vi "state change.vi"(11 "game state":T1(ring)) -> (3 "T/F":bool)   [LabVIEW 2023]
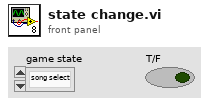
[diagram p1: front panel]
types:
  T1 = enum16{"song select", "difficulty select", "gameplay", "result"}
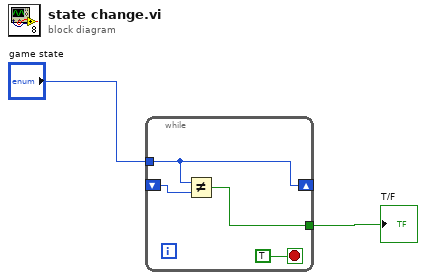
[diagram p0: block diagram]
diagram:
  n1 = while {
    shift-right: [w5] -> _
    shift-left: _ -> [w4]
    tunnel: "game state" -> [w5]
    tunnel: [w3] -> w2
    stop <- TRUE stop-if-true
    n2 = Not Equal?(x=w5, y=w4) -> (x != y?=w3:bool)
  }
  "T/F" <- w2
